vi "Page_Version_Read.vi"(6 "ctlReferences":T1, 8 "error in (no error)":errorcluster, 11 "Class in":refnum<class "IB_MSI.lvclass">) -> (0 "error out":errorcluster, 3 "Class out":refnum<class "IB_MSI.lvclass">)   [LabVIEW 2020, in "IB_MSI.lvclass"]
uses:
  <vilib>/AppBuilder/IB_Classes/MSI/IB_MSI.lvclass
  <resource>/Framework/Providers/Builds/Installer/Pages/controls/IB_UI_Page_Version_Info_References.ctl
  <resource>/Framework/Providers/Builds/Installer/CDK_sTypeDef_ProductVersion.ctl
  <vilib>/AppBuilder/IB_Classes/MSI/IB_MSI.lvclass/IB_MSI.ctl
  <vilib>/AppBuilder/IB_Classes/Installer/Installer.lvclass
panel:
  # "."
  # "."
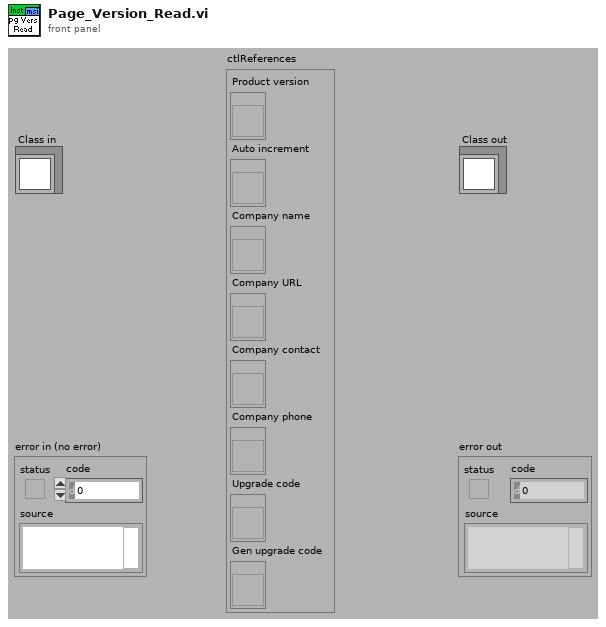
[diagram p1: front panel]
types:
  T1 = typedef "IB_UI_Page_Version_Info_References.ctl" = cluster{"Product version":refnum<vi>, "Auto increment":refnum<vi>, "Company name":refnum<vi>, "Company URL":refnum<vi>, "Company contact":refnum<vi>, "Company phone":refnum<vi>, "Upgrade code":refnum<vi>, "Gen upgrade code":refnum<vi>}
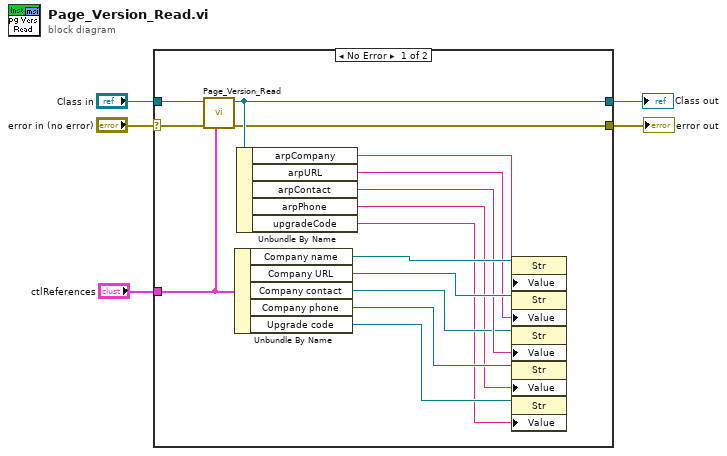
[diagram p0: block diagram]
diagram:
  n1 = case shown="No Error" "error in (no error)" {
    selector: "error in (no error)" -> [w16 w22]
    tunnel: [w15 w22] -> w4
    tunnel: [w17 w21] -> w2
    tunnel: "Class in" -> [w18 w21]
    tunnel: "ctlReferences" -> [w14 _]
    frame No Error {
      n2 = call-parent "Page_Version_Read.vi"("ctlReferences"=w14, "error in (no error)"=w16, "Class in"=w18) -> ("error out"=w15:errorcluster, "Class out"=w17:refnum<class "IB_MSI.lvclass">)  [unwired: 7 out]
      n3 = Unbundle By Name(w14) -> ("Company name"=w20:refnum<vi>, "Company URL"=w13:refnum<vi>, "Company contact"=w10:refnum<vi>, "Company phone"=w9:refnum<vi>, "Upgrade code"=w8:refnum<vi>)
      n4 = Unbundle By Name(w17) -> ("arpCompany"=w19:string, "arpURL"=w12:string, "arpContact"=w11:string, "arpPhone"=w7:string, "upgradeCode"=w6:string)
      n5 = property class="Str"(reference=w20, "Value"=w19) -> ()  [unwired: 1 in, 2 out]
      n6 = property class="Str"(reference=w13, "Value"=w12) -> ()  [unwired: 1 in, 2 out]
      n7 = property class="Str"(reference=w10, "Value"=w11) -> ()  [unwired: 1 in, 2 out]
      n8 = property class="Str"(reference=w9, "Value"=w7) -> ()  [unwired: 1 in, 2 out]
      n9 = property class="Str"(reference=w8, "Value"=w6) -> ()  [unwired: 1 in, 2 out]
    }
    frame Error {
    }
  }
  "error out" <- w4
  "Class out" <- w2
